vi "Destroy.vi"(8 "error in (no error)":errorcluster, 11 "Thread":refnum<class "Thread.lvclass">) -> (0 "error out":errorcluster, 3 "Thread type":refnum<class "Thread.lvclass">)   [LabVIEW 2021, in "DSF Core.lvlib" / "Thread.lvclass"]
uses:
  Thread.lvclass
  Thread.lvclass/Thread.ctl
  <vilib>/NI/Memory Manager/Classes/Pointer/Pointer.lvclass/Pointer.ctl
  <vilib>/NI/Memory Manager/Classes/Pointer/Read.vi
  <vilib>/NI/Memory Manager/Classes/Pointer/Read U8.vi
  <vilib>/NI/Memory Manager/Classes/Pointer/Deallocate.vi
  <vilib>/NI/Memory Manager/Classes/Pointer/Read (No Check).vi
  <vilib>/NI/Memory Manager/Classes/Pointer/Read (No Check) U8.vi
  <vilib>/NI/Memory Manager/Classes/Pointer/Check Move.vi
  <vilib>/NI/Memory Manager/Classes/Pointer/Get Internal.vi
  <vilib>/NI/Memory Manager/Classes/Pointer/Errors.vi
  <vilib>/NI/Memory Manager/Classes/Pointer/Zone.vi
  <vilib>/NI/Memory Manager/Classes/Pointer/Set Address.vi
  <vilib>/NI/Memory Manager/Classes/Pointer/Set Size.vi
  <vilib>/NI/Memory Manager/Classes/Pointer/Set Internal.vi
  <vilib>/NI/Memory Manager/Classes/Pointer/Get Address.vi
  <vilib>/NI/Memory Manager/Classes/Pointer/Check Null Pointer.vi
  <vilib>/NI/Memory Manager/Classes/Pointer/Check Count.vi
  <vilib>/NI/Memory Manager/Classes/Pointer/Check Bounds (Power of 2).vi
  <vilib>/NI/Memory Manager/Classes/Pointer/Create Error.vi
  <vilib>/NI/Memory Manager/Classes/Pointer/Null Pointer.vi
  <vilib>/NI/Memory Manager/Classes/Pointer/Is Null.vi
  <vilib>/NI/Memory Manager/Classes/Pointer/Get Size.vi
  <vilib>/NI/Memory Manager/Classes/Pointer/Out of Bounds.vi
  <vilib>/NI/Memory Manager/Classes/Pointer/Check Bounds.vi
  <vilib>/NI/Memory Manager/VIs/New Error Cluster.vi
  <vilib>/NI/Memory Manager/VIs/New Error Cluster (512B).vi
  <vilib>/NI/Memory Manager/VIs/Set Error Status.vi
  <vilib>/NI/Memory Manager/VIs/Set Error Code.vi
  <vilib>/NI/Memory Manager/VIs/Set Error Source.vi
  <vilib>/NI/Memory Manager/Constants/Constants.vi
  <vilib>/NI/Memory Manager/Constants/Library Name.vi
  <vilib>/NI/Memory Manager/Classes/Pointer/Pointer Error Info.vi
  <vilib>/NI/Memory Manager/VIs/Write String to Source.vi
  <vilib>/NI/Memory Manager/Constants/Pointer Class Name.vi
  <vilib>/NI/Memory Manager/Classes/Pointer/Write Pointer Size to Error.vi
  <vilib>/NI/Memory Manager/VIs/Write Numeric to Source.vi
  <vilib>/NI/Memory Manager/VIs/Write Numeric Scalar to Source (Base10 U64).vi
  <vilib>/NI/Memory Manager/Classes/Pointer/Check Bounds (Pointer).vi
  <vilib>/NI/Memory Manager/Classes/Pointer/Check Bounds (Buffer).vi
  <vilib>/NI/Memory Manager/Classes/Pointer/Buffer Underflow.vi
  Pointers/Error/Error Pointer.lvclass
  C:/Program Files/National Instruments/LabVIEW 2021/vi.lib/NI/Memory Manager/Classes/Pointer/Pointer.lvclass
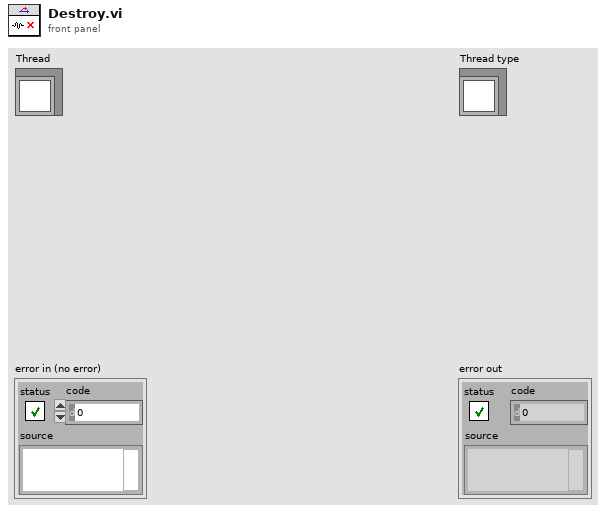
[diagram p1: front panel]
types:
  T1 = typedef "DSF Core.lvlib/Thread.lvclass/Thread State.ctl" = enum8{"Idle", "Running", "Error", "Shut Down"}
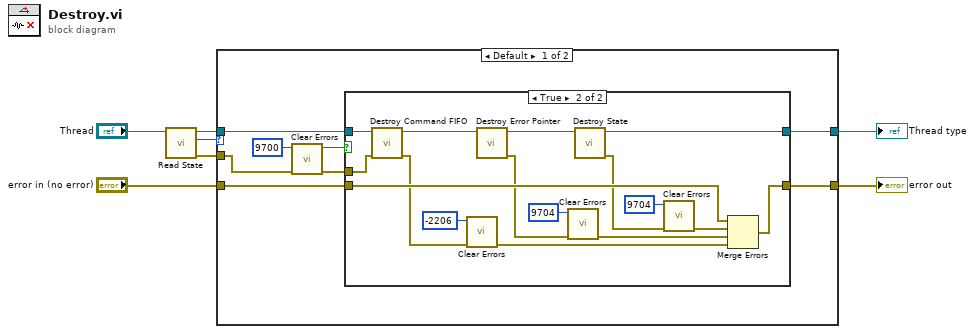
[diagram p0: block diagram]
diagram:
  n1 = call "Read State.vi"("Thread in"="Thread") -> ("error out"=w1:errorcluster, "state"=w2:T1, "Thread out"=w3:refnum<class "Thread.lvclass">)  [unwired: 8 in]
  n2 = case shown="Default" w2 {
    tunnel: "error in (no error)" -> [w15 w34]
    tunnel: [w14 w34] -> w6
    tunnel: [w13 w35] -> w5
    tunnel: w3 -> [w12 w35]
    tunnel: w1 -> [w9 _]
    frame Default {
      n3 = call <vilib>:"Clear Errors.vi"("error in (no error)"=w9, "specific error code to clear (0: all)"=9700) -> ("error out"=w8:errorcluster, "specific error cleared?"=w10:bool)  [unwired: 4 in]
      n4 = case shown="True" w10 {
        tunnel: w15 -> [w16 w33]
        tunnel: [w16 w32] -> w14
        tunnel: [w17 w25] -> w13
        tunnel: w12 -> [w17 w19]
        tunnel: w8 -> [_ w18]
        frame False {
        }
        frame True {
          n5 = call "Destroy Command FIFO.vi"("error in (no error)"=w18, "Thread in"=w19) -> ("error out"=w20:errorcluster, "Thread out"=w31:refnum<class "Thread.lvclass">)  [unwired: 8 in]
          n6 = call <vilib>:"Clear Errors.vi"("error in (no error)"=w20, "specific error code to clear (0: all)"=-2206) -> ("error out"=w21:errorcluster)  [unwired: 4 in, 1 out]
          n7 = call "Destroy Error Pointer.vi"("Thread in"=w31) -> ("error out"=w29:errorcluster, "Thread out"=w26:refnum<class "Thread.lvclass">)  [unwired: 9 in]
          n8 = call <vilib>:"Clear Errors.vi"("error in (no error)"=w29, "specific error code to clear (0: all)"=9704) -> ("error out"=w23:errorcluster)  [unwired: 4 in, 1 out]
          n9 = call "Destroy State.vi"("Thread in"=w26) -> ("error out"=w27:errorcluster, "Thread out"=w25:refnum<class "Thread.lvclass">)  [unwired: 9 in]
          n10 = call <vilib>:"Clear Errors.vi"("error in (no error)"=w27, "specific error code to clear (0: all)"=9704) -> ("error out"=w24:errorcluster)  [unwired: 4 in, 1 out]
          n11 = Merge Errors(w33, w24, w23, w21) -> (w32:errorcluster)
        }
      }
    }
    frame "Shut Down" {
    }
  }
  "error out" <- w6
  "Thread type" <- w5
